vi "Get Base Address.vi"(6 "offset":i32, 8 "error in (no error)":errorcluster, 11 "bitfile xml in":string) -> (0 "error out":errorcluster, 2 "value":u32)   [LabVIEW 2010, in "FPGA Bitfile Utility.lvlib"]
uses:
  <userlib>/_FPGA Interface Advanced Tools/FPGA Bitfile Utility/FPGA Bitfile Utility.lvlib
  <vilib>/rvi/Utilities/XML/nirviXML_GetValue_String.vi
  <vilib>/rvi/Utilities/XML/nirviXML_GetValue_U32.vi
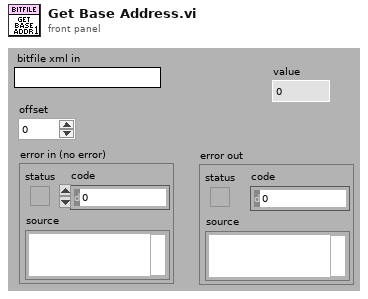
[diagram p1: front panel]
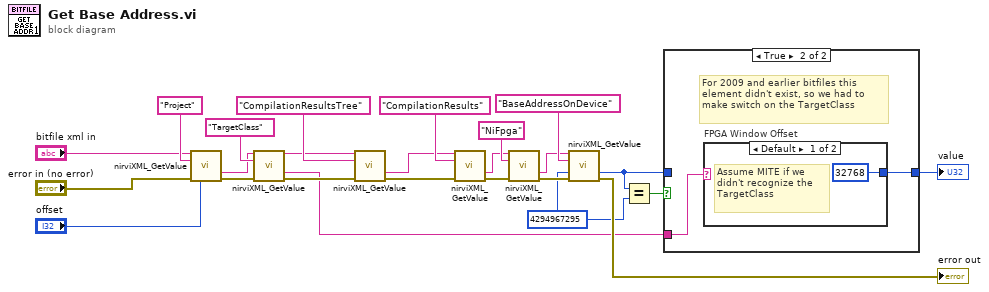
[diagram p0: block diagram]
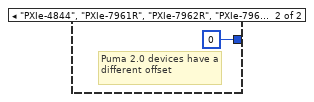
[diagram p3: hidden frame]
diagram:
  w4 = u32 4294967295
  n1 = call-poly <vilib>:"nirviXML_GetValue.vi"("xml string in"="bitfile xml in", "tag name in"="Project" ("Element"), "error in (no error)"="error in (no error)", "offset"="offset") -> ("value"=w12:string, "error out"=w11:errorcluster)  [unwired: 1 in, 9 out]
  n2 = call-poly <vilib>:"nirviXML_GetValue.vi"("xml string in"=w12, "tag name in"="TargetClass" ("Element"), "error in (no error)"=w11) -> ("xml string out"=w9:string, "value"=w2:string, "error out"=w8:errorcluster)  [unwired: 2 in, 8 out]
  n3 = call-poly <vilib>:"nirviXML_GetValue.vi"("xml string in"=w9, "tag name in"="CompilationResultsTree" ("Element"), "error in (no error)"=w8) -> ("value"=w7:string, "error out"=w6:errorcluster)  [unwired: 2 in, 9 out]
  n4 = call-poly <vilib>:"nirviXML_GetValue.vi"("xml string in"=w7, "tag name in"="CompilationResults" ("Element"), "error in (no error)"=w6) -> ("value"=w20:string, "error out"=w19:errorcluster)  [unwired: 2 in, 9 out]
  n5 = call-poly <vilib>:"nirviXML_GetValue.vi"("xml string in"=w20, "tag name in"="NiFpga" ("Element"), "error in (no error)"=w19) -> ("value"=w23:string, "error out"=w22:errorcluster)  [unwired: 2 in, 9 out]
  n6 = call-poly <vilib>:"nirviXML_GetValue.vi"("xml string in"=w23, "tag name in"="BaseAddressOnDevice" ("Element"), "default value"=w4, "error in (no error)"=w22) -> ("value"=w5:u32, "error out"=→"error out":errorcluster)  [unwired: 1 in, 9 out]
  n7 = Equal?(x=w5, y=w4) -> (x = y?=w3:bool)
  n8 = case shown="True" w3 {
    tunnel: w2 -> [_ w28]
    tunnel: [w26 w27] -> w1
    tunnel: w5 -> [w26 _]
    frame False {
      # "If we successfully got something legitimate, simply use it"
    }
    frame True {
      # "For 2009 and earlier bitfiles this element didn't exist, so we had to make switch on the TargetClass"
      n9 = case "FPGA Window Offset" shown="Default" w28 {
        tunnel: [u32 32768 u32 0] -> w27
        frame Default {
          # "Assume MITE if we didn't recognize the TargetClass"
        }
        frame "PXIe-4844", "PXIe-7961R", "PXIe-7962R", "PXIe-7965R" {
          # "Puma 2.0 devices have a different offset"
        }
      }
    }
  }
  "value" <- w1
